vi "Copy Firmware Libraries.vi"(8 "Error In":errorcluster, 11 "Library Destination Dir":path=path "C:/Program Files (x86)/National Instruments/LabVIEW 2011/vi.lib/LabVIEW Hacker/LINX/Firmware/Source/librariestest") -> (0 "Error Out":errorcluster)   [LabVIEW 2020, in "LMH-LINX.lvlib"]
uses:
  <vilib>/MakerHub/LINX/LMH-LINX.lvlib
  <vilib>/MakerHub/LINX/Private/Type Defs/Firmware Library Component.ctl
  <vilib>/Utility/config.llb/Read Key (String).vi
  <vilib>/Utility/config.llb/NI_LVConfig.lvlib
  <vilib>/MakerHub/Toolbox/LMH-Toolbox.lvlib
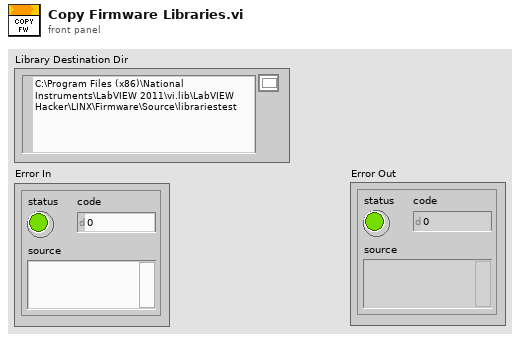
[diagram p1: front panel]
types:
  T1 = typedef "NI_LVConfig.lvlib/Config Data RefNum.ctl" = refnum<k1>
  T2 = typedef "LMH-LINX.lvlib/Firmware Library Component.ctl" = cluster{"Source":path, "Destination":path}
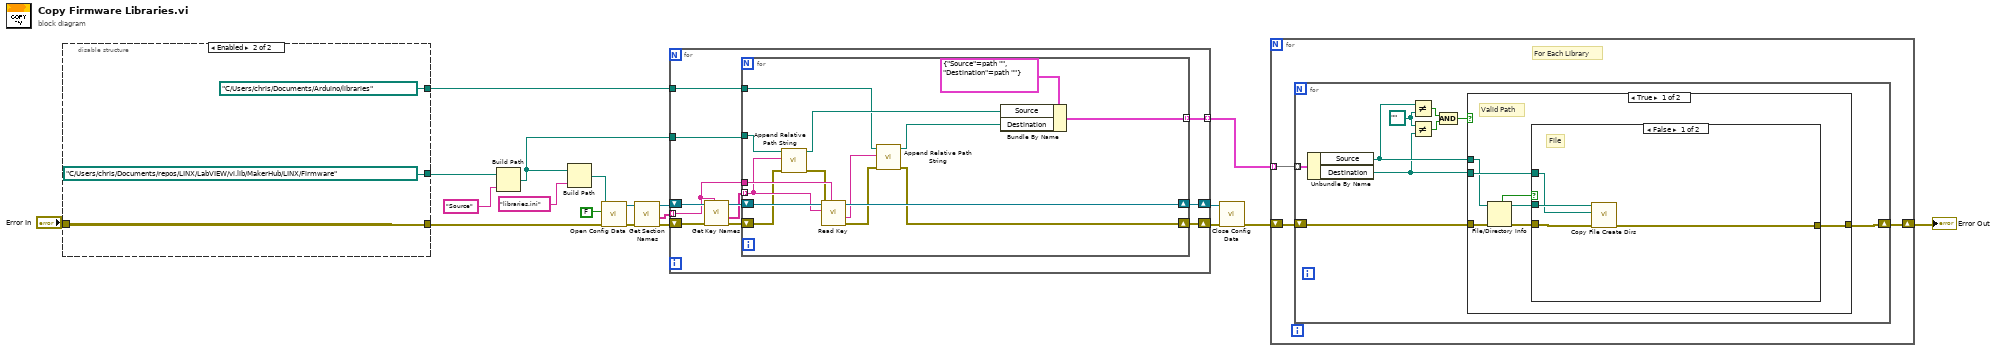
[diagram p0: block diagram]
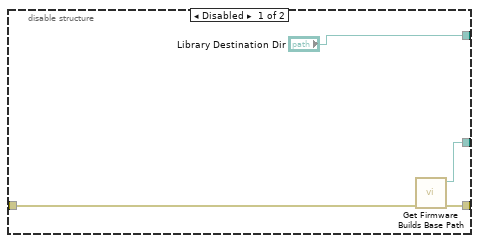
[diagram p2: hidden frame]
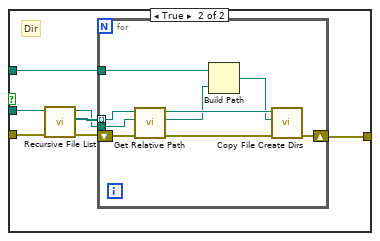
[diagram p3: hidden frame]
diagram:
  n1 = disable-structure shown="Enabled" {
    disable-tunnel: "Error In" -> [w23 w26]
    disable-tunnel: [w22 w26] -> w3
    disable-tunnel: [w21 path "C:/Users/chris/Documents/repos/LINX/LabVIEW/vi.lib/MakerHub/LINX/Firmware" ("Firmware Builds Base Path")] -> w2
    disable-tunnel: ["Library Destination Dir" path "C:/Users/chris/Documents/Arduino/libraries" ("Library Destination Dir")] -> w1
    frame Disabled {
      n2 = call <vilib>:"Get Firmware Builds Base Path.vi"("Error In"=w23) -> ("Error Out"=w22:errorcluster, "Firmware Builds Base Path"=w21:path)  [unwired: 9 in]
    }
    frame Enabled {
    }
  }
  n3 = Build Path(base path=w2, name or relative path="Source") -> (appended path=w4:path)
  n4 = Build Path(base path=w4, name or relative path="libraries.ini") -> (appended path=w8:path)
  n5 = call <vilib>:"Open Config Data.vi"("error in (no error)"=w3, "create file if necessary (T)"=FALSE, "configuration file path"=w8) -> ("error out"=w18:errorcluster, "refnum"=w19:T1)  [unwired: 6 in, 1 out]
  n6 = call <vilib>:"Get Section Names.vi"("error in (no error)"=w18, "refnum"=w19) -> ("error out"=w14:errorcluster, "section names"=w12:string[], "refnum out"=w16:T1)  [unwired: 7 in]
  n7 = for {
    shift-right: [w34] -> w15
    shift-left: w16 -> [w37]
    shift-right: [w32] -> w13
    shift-left: w14 -> [w36]
    tunnel: w12 -> [w30] mode=indexing
    tunnel: w4 -> [w29]
    tunnel: [w28] -> w11 mode=indexing
    tunnel: w1 -> [w27]
    n8 = call <vilib>:"Get Key Names.vi"("section"=w30, "error in (no error)"=w36, "refnum"=w37) -> ("error out"=w33:errorcluster, "key names"=w31:string[], "refnum out"=w35:T1)  [unwired: 5 in, 1 out]
    n9 = for {
      shift-right: [w51] -> w34
      shift-left: w35 -> [w52]
      shift-right: [w42] -> w32
      shift-left: w33 -> [w44]
      tunnel: w31 -> [w45] mode=indexing
      tunnel: w30 -> [w50]
      tunnel: w29 -> [w46]
      tunnel: [w39] -> w28 mode=indexing
      tunnel: w27 -> [w38]
      n10 = call <vilib>:"Append Relative Path String.vi"("Error In"=w44, "Relative Path"=w45, "Base Path"=w46) -> ("Error Out"=w43:errorcluster, "Absolute Path"=w41:path)  [unwired: 7 in]
      n11 = call-poly <vilib>:"Read Key.vi"("section"=w50, "error in (no error)"=w43, "key"=w45, "refnum"=w52) -> ("error out"=w49:errorcluster, "value"=w48:string, "refnum out"=w51:T1)  [unwired: 4 in, 1 out]
      n12 = call <vilib>:"Append Relative Path String.vi"("Error In"=w49, "Relative Path"=w48, "Base Path"=w38) -> ("Error Out"=w42:errorcluster, "Absolute Path"=w40:path)  [unwired: 7 in]
      n13 = Bundle By Name(cluster=T2 {"Source"=path "", "Destination"=path ""} ("Library Component"), "Source"=w41, "Destination"=w40) -> (w39:T2)
    }
  }
  n14 = call <vilib>:"Close Config Data.vi"("error in (no error)"=w13, "refnum"=w15) -> ("error out"=w10:errorcluster)  [unwired: 8 in, 1 out]
  n15 = for {
    tunnel: w11 -> [w54] mode=indexing
    shift-right: [w53] -> w9
    shift-left: w10 -> [w55]
    # "For Each Library"
    n16 = for {
      tunnel: w54 -> [w64] mode=indexing
      shift-right: [w63] -> w53
      shift-left: w55 -> [w56]
      w60 = path ""
      n17 = Unbundle By Name(w64) -> ("Source"=w59:path, "Destination"=w58:path)
      n18 = Not Equal?(x=w59, y=w60) -> (x != y?=w62:bool)
      n19 = Not Equal?(x=w60, y=w58) -> (x != y?=w61:bool)
      n20 = And(x=w62, y=w61) -> (x .and. y?=w57:bool)
      n21 = case shown="True" w57 {
        tunnel: [w70 w92] -> w63
        tunnel: w58 -> [w71 _]
        tunnel: w59 -> [w68 _]
        tunnel: w56 -> [w69 w92]
        frame True {
          # "Valid Path"
          n22 = File/Directory Info(path=w68, error in=w69) -> (path out=w67:path, directory=w65:bool, error out=w66:errorcluster)  [unwired: 4 out]
          n23 = case shown="False" w65 {
            tunnel: w71 -> [w73 w79]
            tunnel: [w72 w78] -> w70
            tunnel: w67 -> [w74 w77]
            tunnel: w66 -> [w75 w76]
            frame False {
              # "File"
              n24 = call <vilib>:"Copy File Create Dirs.vi"("Error In"=w75, "Destination"=w73, "Source"=w74) -> ("Error Out"=w72:errorcluster)  [unwired: 8 in]
            }
            frame True {
              # "Dir"
              n25 = call <vilib>:"Recursive File List.vi"("error in (no error)"=w76, "Folder Path"=w77) -> ("error out"=w82:errorcluster, "All Files in Dir"=w81:path[], "dup Folder Path"=w80:path)  [unwired: 5 in, 2 out]
              n26 = for {
                tunnel: w81 -> [w90] mode=indexing
                tunnel: w80 -> [w89]
                tunnel: w79 -> [w86]
                shift-right: [w83] -> w78
                shift-left: w82 -> [w91]
                n27 = call <vilib>:"Get Relative Path.vi"("Error In"=w91, "Relative Path Root"=w89, "File / Folder"=w90) -> ("Error Out"=w88:errorcluster, "Relative Path"=w85:path, "Duplicate File / Folder"=w87:path)  [unwired: 6 in]
                n28 = Build Path(base path=w86, name or relative path=w85) -> (appended path=w84:path)
                n29 = call <vilib>:"Copy File Create Dirs.vi"("Error In"=w88, "Destination"=w84, "Source"=w87) -> ("Error Out"=w83:errorcluster)  [unwired: 8 in]
              }
            }
          }
        }
        frame False {
          # "Invalid Path"
        }
      }
    }
  }
  "Error Out" <- w9
